vi "pixel counter z.vi"(8 "counter cluster in":T2, 9 "scanning":bool, 10 "scan specification":T3, 11 "tag lens trigger":bool) -> (0 "counter cluster out":T2, 1 "trigger diagnostics":T1, 2 "fly back":bool, 3 "acquire":bool, 4 "new line":bool)   [LabVIEW 2010]
uses:
  scan_specification_tagResonant.ctl
  counter_cluster_tagResonant.ctl
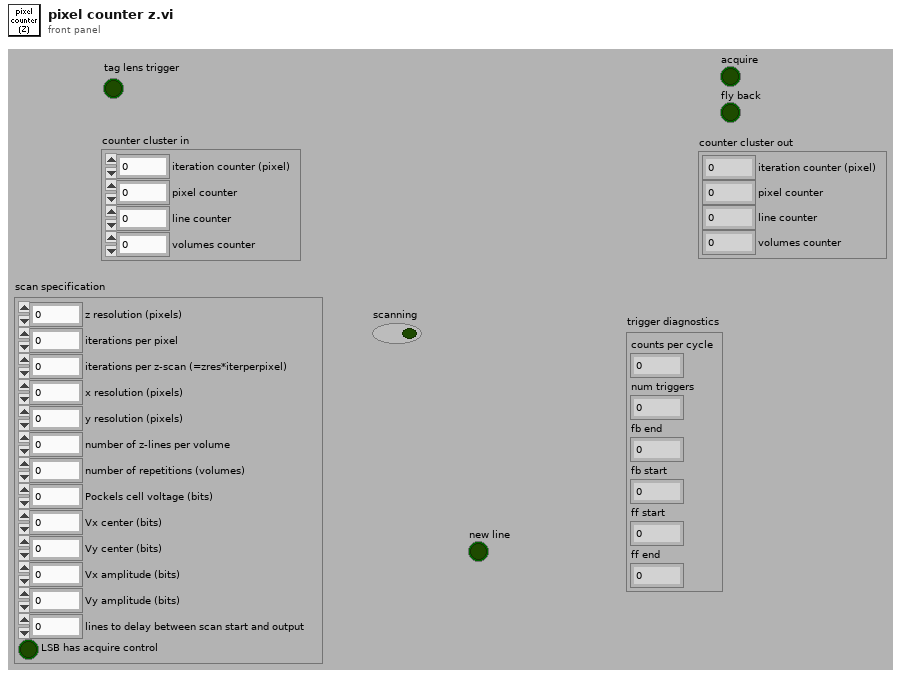
[diagram p1: front panel]
types:
  T1 = cluster{"counts per cycle":u16, "num triggers":u32, "fb end":u16, "fb start":u16, "ff start":u16, "ff end":u16}
  T2 = typedef "counter_cluster_tagResonant.ctl" = cluster{"iteration counter (pixel)":u16, "pixel counter":u16, "line counter":i16, "volumes counter":u16}
  T3 = typedef "scan_specification_tagResonant.ctl" = cluster{"z resolution (pixels)":u16, "iterations per pixel":u16, "iterations per z-scan (=zres*iterperpixel)":u16, "x resolution (pixels)":u16, "y resolution (pixels)":u16, "number of z-lines per volume":u16, "number of repetitions (volumes)":i32, "Pockels cell voltage (bits)":i16, "Vx center (bits)":i16, "Vy center (bits)":i16, "Vx amplitude (bits)":i16, "Vy amplitude (bits)":i16, "lines to delay between scan start and output":u16, "LSB has acquire control":bool}
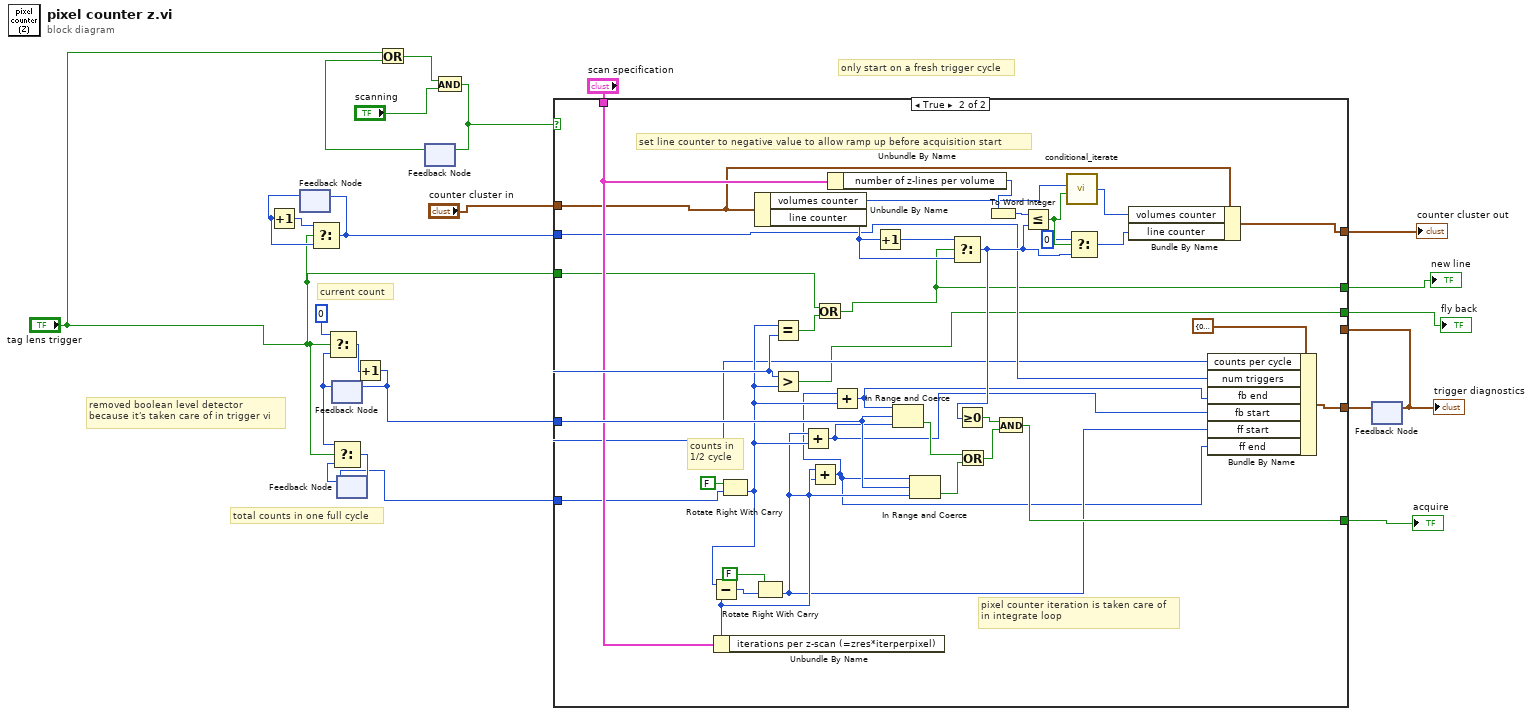
[diagram p0: block diagram]
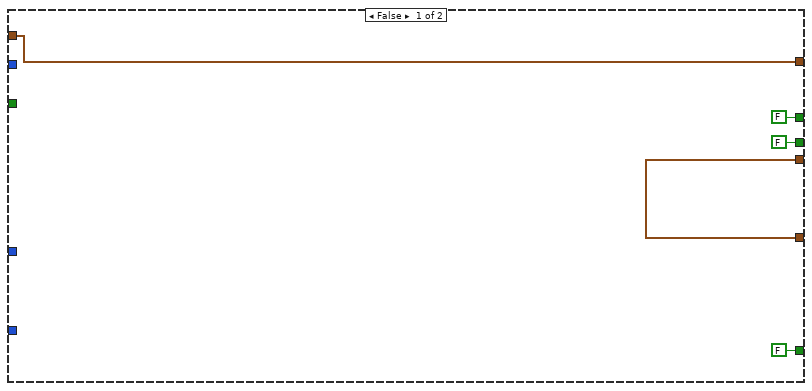
[diagram p2: hidden frame]
diagram:
  # "removed boolean level detector\nbecause it's taken care of in trigger vi"
  # "only start on a fresh trigger cycle"
  # "total counts in one full cycle"
  # "current count"
  n1 = feedback #1() -> (w13:u32)  [unwired: 1 in]
  n2 = Increment(x=w13) -> (x+1=w14:u32)
  n3 = Select(t=w14, s="tag lens trigger", f=w13) -> (s? t:f=w12:u32)
  n4 = feedback-in #1(w12) -> ()
  n5 = feedback #2() -> (w20:u16)  [unwired: 1 in]
  n6 = Select(t=u16 0, s="tag lens trigger", f=w20) -> (s? t:f=w21:u16)
  n7 = feedback #3() -> (w11:u16)  [unwired: 1 in]
  n8 = Select(t=w20, s="tag lens trigger", f=w11) -> (s? t:f=w19:u16)
  n9 = feedback-in #3(w19) -> ()
  n10 = Increment(x=w21) -> (x+1=w18:u16)
  n11 = feedback-in #2(w18) -> ()
  n12 = feedback #4() -> (w8:bool)  [unwired: 1 in]
  n13 = Or(x="tag lens trigger", y=w8) -> (x .or. y?=w9:bool)
  n14 = And(x=w9, y="scanning") -> (x .and. y?=w7:bool)
  n15 = feedback-in #4(w7) -> ()
  n16 = feedback #5() -> (w4:T1)  [unwired: 1 in]
  "trigger diagnostics" <- w4
  n17 = case shown="True" w7 {
    tunnel: w18 -> [_ w57]
    tunnel: "scan specification" -> [_ w54]
    tunnel: [w27 w48] -> w16
    tunnel: [FALSE w40] -> w15
    tunnel: "tag lens trigger" -> [_ w39]
    tunnel: w12 -> [_ w37]
    tunnel: w11 -> [_ w36]
    tunnel: [w25 w31] -> w5
    tunnel: "counter cluster in" -> [w27 w30]
    tunnel: w4 -> [w25 _]
    tunnel: [FALSE w29] -> w2
    tunnel: [FALSE w28] -> w1
    frame False {
    }
    frame True {
      # "set line counter to negative value to allow ramp up before acquisition start"
      # "pixel counter iteration is taken care of\nin integrate loop"
      # "counts in \n1/2 cycle"
      n18 = Unbundle By Name(w54) -> ("iterations per z-scan (=zres*iterperpixel)"=w58:u16)
      n19 = Rotate Right With Carry(2:w36, 3:FALSE ("carry")) -> (0:w56:u16)  [unwired: 1 out]
      n20 = Subtract(x=w56, y=w58) -> (x-y=w62:u16)
      n21 = Unbundle By Name(w30) -> ("volumes counter"=w51:u16, "line counter"=w47:i16)
      n22 = Rotate Right With Carry(2:w62, 3:FALSE ("carry")) -> (0:w33:u16)  [unwired: 1 out]
      n23 = Equal?(x=w56, y=w57) -> (x = y?=w55:bool)
      n24 = Greater?(x=w57, y=w56) -> (0:w28:bool)
      n25 = Add(x=w33, y=w56) -> (x+y=w34:u16)
      n26 = Add(x=w58, y=w33) -> (x+y=w32:u16)
      n27 = Or(x=w39, y=w55) -> (x .or. y?=w29:bool)
      n28 = Unbundle By Name(w54) -> ("number of z-lines per volume"=w53:u16)
      n29 = Add(x=w32, y=w56) -> (x+y=w35:u16)
      n30 = Increment(x=w47) -> (x+1=w46:i16)
      n31 = In Range and Coerce(upper limit=w35, x=w57, lower limit=w34) -> (In Range?=w60:bool)  [unwired: 1 out]
      n32 = In Range and Coerce(upper limit=w32, x=w57, lower limit=w33) -> (In Range?=w59:bool)  [unwired: 1 out]
      n33 = Select(t=w46, s=w29, f=w47) -> (s? t:f=w43:i16)
      n34 = Greater Or Equal To 0?(x=w43) -> (x >= 0?=w42:bool)
      n35 = Or(x=w60, y=w59) -> (x .or. y?=w41:bool)
      n36 = To Word Integer(number=w53) -> (16bit integer=w44:i16)
      n37 = And(x=w42, y=w41) -> (x .and. y?=w40:bool)
      n38 = Less Or Equal?(x=w44, y=w43) -> (x <= y?=w52:bool)
      n39 = call "conditional_iterate.vi"("iterate?"=w52, "number in"=w51) -> ("number out"=w50:u16)  [unwired: 4 in]
      n40 = Select(t=i16 0, s=w52, f=w43) -> (s? t:f=w49:i16)
      n41 = Bundle By Name(cluster=w30, "volumes counter"=w50, "line counter"=w49) -> (w48:T2)
      n42 = Bundle By Name(cluster=T1 {"counts per cycle"=0, "num triggers"=0, "fb end"=0, "fb start"=0, "ff start"=0, "ff end"=0} ("trigger diagnostics"), "counts per cycle"=w36, "num triggers"=w37, "fb end"=w35, "fb start"=w34, "ff start"=w33, "ff end"=w32) -> (w31:T1)
    }
  }
  "acquire" <- w15
  "counter cluster out" <- w16
  "new line" <- w2
  "fly back" <- w1
  n43 = feedback-in #5(w5) -> ()
